vi "FPGANic.Read-Debug-FIFOs.vi"(8 "error in":errorcluster, 10 "Value":bool, 11 "Refnum in":refnum<k20>) -> (0 "error out":errorcluster, 3 "Debug Data":T1)   [LabVIEW 2017]
uses:
  <vilib>/Utility/error.llb/Error Cluster From Error Code.vi
  <vilib>/rvi/errors/niLvFpgaAdjustHostInterfaceError.vi
  <vilib>/rvi/interface/nirviMethod/nirviMethod.xnode
  <vilib>/FPGAPlugInAG/Dynamic/niLvFpga_ReadFifo_Dynamic.vi
  <vilib>/rvi/errors/niLvFpgaMergeErrorWithErrorCode.vi
panel:
  out "Debug FIFO 2":u32[](array[numeric])
  out "Debug FIFO 1":u32[](array[numeric])
  out "Read Probe":u64[](array[numeric])
  out "Write Probe 1":u64[](array[numeric])
  out "Write Probe 2":u64[](array[numeric])
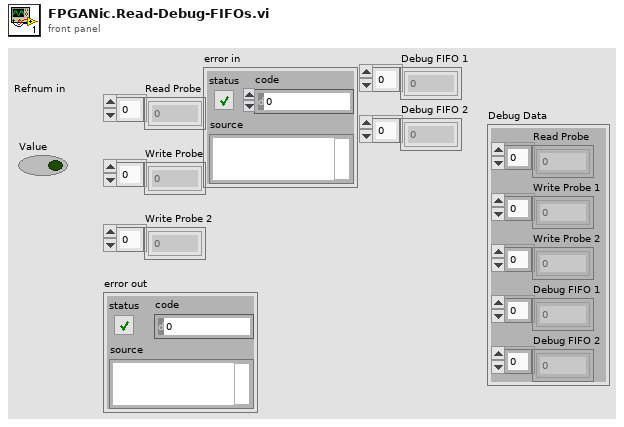
[diagram p1: front panel]
types:
  T1 = cluster{"Read Probe":u64[], "Write Probe 1":u64[], "Write Probe 2":u64[], "Debug FIFO 1":u32[], "Debug FIFO 2":u32[]}
  T2 = cluster{"Data":u64[], "Data":u64[], "Data":u64[], "Data":u32[], "Data":u32[]}
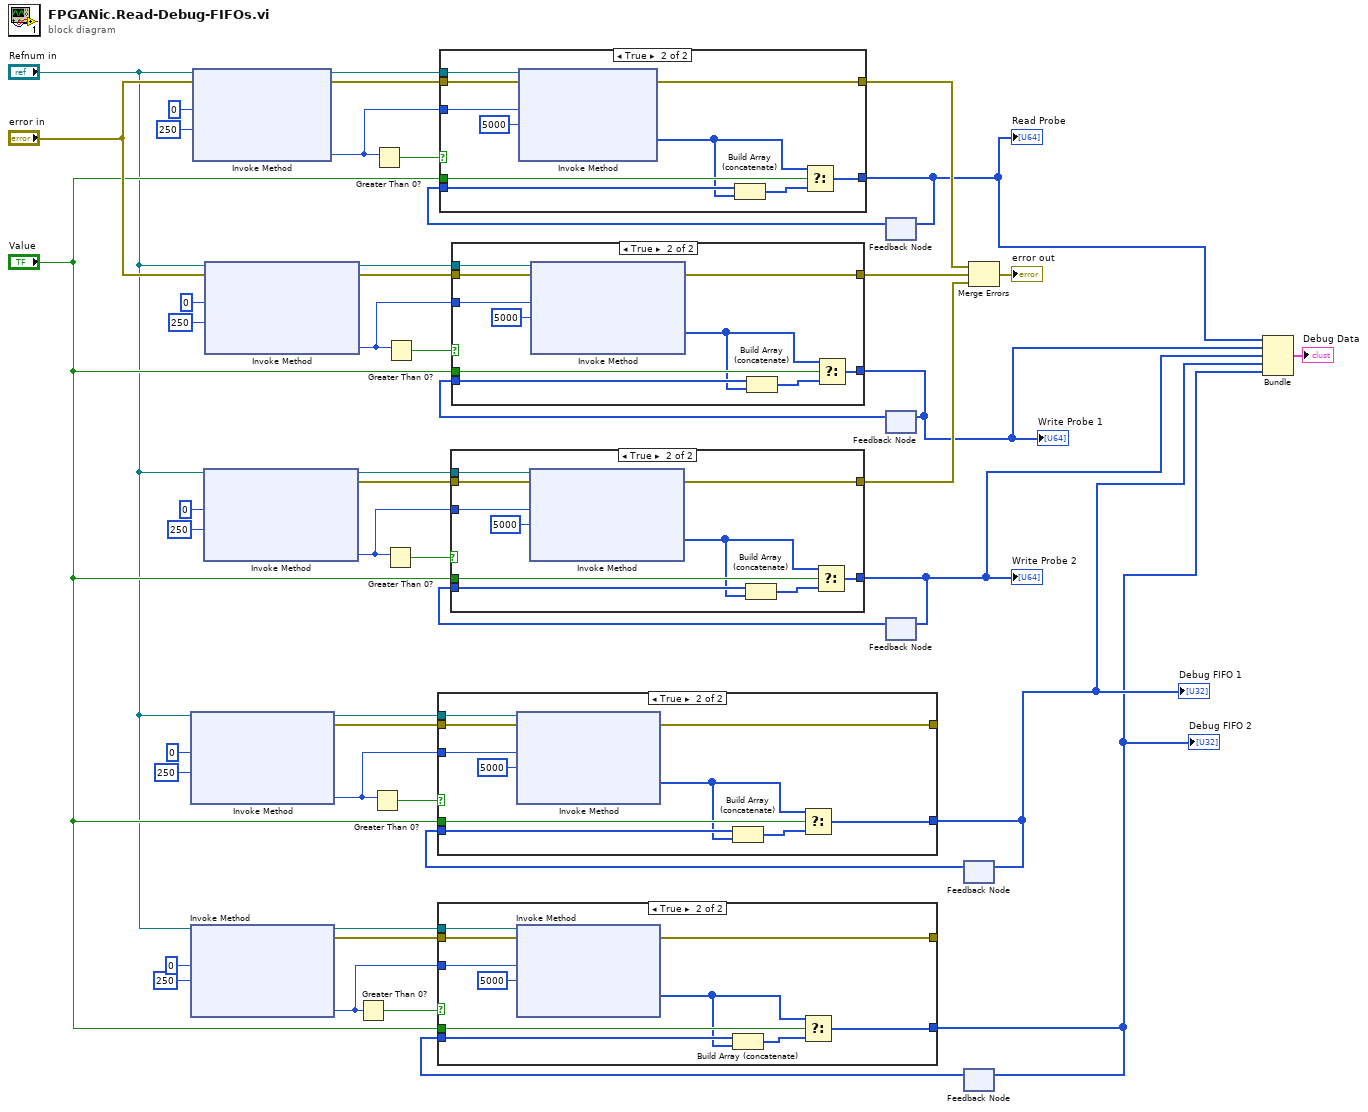
[diagram p0: block diagram]
diagram:
  n1 = xnode "Invoke Method"("FPGA VI Reference In"="Refnum in", "Number of Elements"=u32 0, "Timeout (ms)"=250) -> ("FPGA VI Reference Out"=w17:refnum<k20>, "error out"=w18:errorcluster, "Elements Remaining"=w19:u32)  [unwired: 1 in, 1 out]
  n2 = xnode "Invoke Method"("FPGA VI Reference In"="Refnum in", "Number of Elements"=u32 0, "Timeout (ms)"=250) -> ("FPGA VI Reference Out"=w13:refnum<k20>, "error out"=w12:errorcluster, "Elements Remaining"=w9:u32)  [unwired: 1 in, 1 out]
  n3 = xnode "Invoke Method"("FPGA VI Reference In"="Refnum in", "error in"="error in", "Number of Elements"=u32 0, "Timeout (ms)"=250) -> ("FPGA VI Reference Out"=w29:refnum<k20>, "error out"=w28:errorcluster, "Elements Remaining"=w27:u32)  [unwired: 1 out]
  n4 = xnode "Invoke Method"("FPGA VI Reference In"="Refnum in", "Number of Elements"=u32 0, "Timeout (ms)"=250) -> ("FPGA VI Reference Out"=w43:refnum<k20>, "error out"=w42:errorcluster, "Elements Remaining"=w41:u32)  [unwired: 1 in, 1 out]
  n5 = xnode "Invoke Method"("FPGA VI Reference In"="Refnum in", "error in"="error in", "Number of Elements"=u32 0, "Timeout (ms)"=250) -> ("FPGA VI Reference Out"=w36:refnum<k20>, "error out"=w35:errorcluster, "Elements Remaining"=w34:u32)  [unwired: 1 out]
  n6 = Greater Than 0?(x=w9) -> (x > 0?=w11:bool)
  n7 = Greater Than 0?(x=w19) -> (x > 0?=w20:bool)
  n8 = Greater Than 0?(x=w27) -> (x > 0?=w26:bool)
  n9 = Greater Than 0?(x=w41) -> (x > 0?=w40:bool)
  n10 = Greater Than 0?(x=w34) -> (x > 0?=w33:bool)
  n11 = feedback #1() -> (w30:u64[])  [unwired: 1 in]
  n12 = case shown="True" w26 {
    tunnel: w30 -> [w50 w60]
    tunnel: w27 -> [_ w59]
    tunnel: w28 -> [w49 w57]
    tunnel: w29 -> [_ w56]
    tunnel: [w50 w53] -> w2
    tunnel: [w49 w55] -> w46
    tunnel: "Value" -> [_ w52]
    frame False {
    }
    frame True {
      n13 = xnode "Invoke Method"("FPGA VI Reference In"=w56, "error in"=w57, "Number of Elements"=w59, "Timeout (ms)"=5000) -> ("error out"=w55:errorcluster, "Data"=w51:u64[])  [unwired: 2 out]
      n14 = Build Array (concatenate)(w60, w51) -> (w54:u64[])
      n15 = Select(t=w51, s=w52, f=w54) -> (s? t:f=w53:u64[])
    }
  }
  "Read Probe" <- w2
  n16 = feedback-in #1(w2) -> ()
  n17 = feedback #2() -> (w37:u64[])  [unwired: 1 in]
  n18 = case shown="True" w33 {
    tunnel: w37 -> [w62 w72]
    tunnel: w34 -> [_ w71]
    tunnel: w35 -> [w61 w69]
    tunnel: w36 -> [_ w68]
    tunnel: [w62 w65] -> w6
    tunnel: [w61 w67] -> w47
    tunnel: "Value" -> [_ w64]
    frame False {
    }
    frame True {
      n19 = xnode "Invoke Method"("FPGA VI Reference In"=w68, "error in"=w69, "Number of Elements"=w71, "Timeout (ms)"=5000) -> ("error out"=w67:errorcluster, "Data"=w63:u64[])  [unwired: 2 out]
      n20 = Build Array (concatenate)(w72, w63) -> (w66:u64[])
      n21 = Select(t=w63, s=w64, f=w66) -> (s? t:f=w65:u64[])
    }
  }
  "Write Probe 1" <- w6
  n22 = feedback-in #2(w6) -> ()
  n23 = feedback #3() -> (w44:u64[])  [unwired: 1 in]
  n24 = case shown="True" w40 {
    tunnel: w44 -> [w74 w84]
    tunnel: w41 -> [_ w83]
    tunnel: w42 -> [w73 w81]
    tunnel: w43 -> [_ w80]
    tunnel: [w74 w77] -> w5
    tunnel: [w73 w79] -> w48
    tunnel: "Value" -> [_ w76]
    frame False {
    }
    frame True {
      n25 = xnode "Invoke Method"("FPGA VI Reference In"=w80, "error in"=w81, "Number of Elements"=w83, "Timeout (ms)"=5000) -> ("error out"=w79:errorcluster, "Data"=w75:u64[])  [unwired: 2 out]
      n26 = Build Array (concatenate)(w84, w75) -> (w78:u64[])
      n27 = Select(t=w75, s=w76, f=w78) -> (s? t:f=w77:u64[])
    }
  }
  "Write Probe 2" <- w5
  n28 = feedback-in #3(w5) -> ()
  n29 = feedback #4() -> (w16:u32[])  [unwired: 1 in]
  n30 = case shown="True" w20 {
    tunnel: w16 -> [w86 w96]
    tunnel: w19 -> [_ w95]
    tunnel: w18 -> [w85 w93]
    tunnel: w17 -> [_ w92]
    tunnel: [w86 w89] -> w4
    tunnel: [w85 w91] -> _
    tunnel: "Value" -> [_ w88]
    frame False {
    }
    frame True {
      n31 = xnode "Invoke Method"("FPGA VI Reference In"=w92, "error in"=w93, "Number of Elements"=w95, "Timeout (ms)"=5000) -> ("error out"=w91:errorcluster, "Data"=w87:u32[])  [unwired: 2 out]
      n32 = Build Array (concatenate)(w96, w87) -> (w90:u32[])
      n33 = Select(t=w87, s=w88, f=w90) -> (s? t:f=w89:u32[])
    }
  }
  "Debug FIFO 1" <- w4
  n34 = feedback-in #4(w4) -> ()
  n35 = feedback #5() -> (w10:u32[])  [unwired: 1 in]
  n36 = case shown="True" w11 {
    tunnel: w10 -> [w98 w108]
    tunnel: w9 -> [_ w107]
    tunnel: w12 -> [w97 w105]
    tunnel: w13 -> [_ w104]
    tunnel: [w98 w101] -> w3
    tunnel: [w97 w103] -> _
    tunnel: "Value" -> [_ w100]
    frame False {
    }
    frame True {
      n37 = xnode "Invoke Method"("FPGA VI Reference In"=w104, "error in"=w105, "Number of Elements"=w107, "Timeout (ms)"=5000) -> ("error out"=w103:errorcluster, "Data"=w99:u32[])  [unwired: 2 out]
      n38 = Build Array (concatenate)(w108, w99) -> (w102:u32[])
      n39 = Select(t=w99, s=w100, f=w102) -> (s? t:f=w101:u32[])
    }
  }
  "Debug FIFO 2" <- w3
  n40 = feedback-in #5(w3) -> ()
  n41 = Merge Errors(w46, w47, w48) -> (→"error out":errorcluster)
  n42 = Bundle("Data"=w2, "Data"=w6, "Data"=w5, "Data"=w4, "Data"=w3) -> (→"Debug Data":T2)  [unwired: 1 in]
